vi "FilterCustomDeviceVIs.vi"(8 "error in (no error)":errorcluster, 11 "custom device VIs in":T2(array[cluster])) -> (0 "error out":errorcluster, 3 "custom device VIs out":T1(array[cluster]))   [LabVIEW 2017, in "VeriStandTestUtilities.lvlib"]
uses:
  VeriStandTestUtilities.lvlib
  NationalInstruments.VeriStand.XMLReader
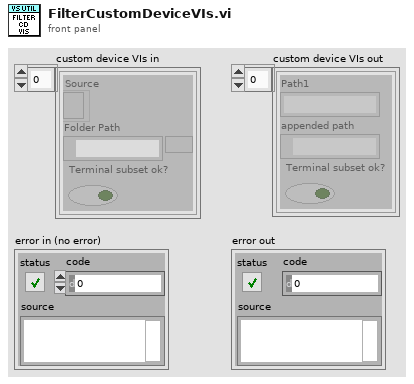
[diagram p1: front panel]
types:
  T1 = cluster{"Path1":string, "appended path":path, "Terminal subset ok?":bool}[]
  T2 = cluster{"Source":refnum<k24>, "Folder Path":path, "Terminal subset ok?":bool}[]
  T3 = cluster{"Path1":string, "appended path":path, "Terminal subset ok?":bool}
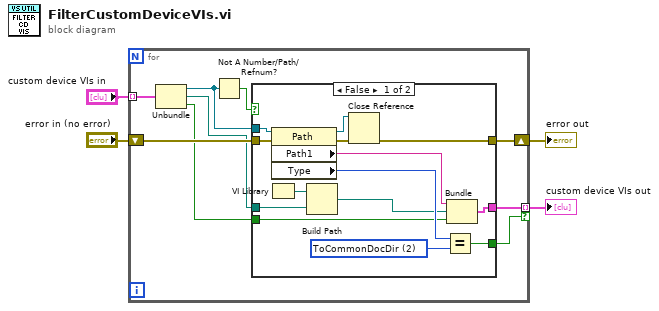
[diagram p0: block diagram]
diagram:
  n1 = for {
    tunnel: "custom device VIs in" -> [w13] mode=indexing
    shift-right: [w10] -> w2
    shift-left: "error in (no error)" -> [w8]
    tunnel: [w6] -> w1 mode=indexing if=w9
    n2 = Unbundle(w13) -> ("Source"=w11:refnum<k24>, "Folder Path"=w7:path, "Terminal subset ok?"=w5:bool)
    n3 = Not A Number/Path/Refnum?(number/path/refnum=w11) -> (NaN/Path/Refnum?=w12:bool)
    n4 = case shown="False" w12 {
      tunnel: w11 -> [w27 _]
      tunnel: [w24 _] -> w9
      tunnel: [w21 w28] -> w10
      tunnel: w8 -> [w20 w28]
      tunnel: w7 -> [w19 _]
      tunnel: [w15 _] -> w6
      tunnel: w5 -> [w14 _]
      frame False {
        w25 = 2 items=["Absolute", "ToBase", "ToCommonDocDir", "ToApplicationDataDir"] ("Type")
        n5 = VI Library() -> (path=w18:path)
        n6 = property class="Path"(reference=w27, error in=w20) -> (reference out=w23:refnum<k24>, error out=w22:errorcluster, "Path1"=w16:string, "Type"=w26:i32)
        n7 = Build Path(base path=w18, name or relative path=w19) -> (appended path=w17:path)
        n8 = Close Reference(reference=w23, error in (no error)=w22) -> (error out=w21:errorcluster)
        n9 = Equal?(x=w26, y=w25) -> (x = y?=w24:bool)
        n10 = Bundle("Path1"=w16, "appended path"=w17, "Terminal subset ok?"=w14) -> (w15:T3)  [unwired: 1 in]
      }
      frame True {
      }
    }
  }
  "error out" <- w2
  "custom device VIs out" <- w1
